vi "7AM.vi"() -> ()   [LabVIEW 2013]
uses:
  <vilib>/measure/NI_MABase.lvlib
panel:
  out "Filtered Signal":dynamicdata(graph)
  in  "sampling info 3":cluster{"Fs":dbl, "#s":dbl}={"Fs"=1000.0, "#s"=1000.0} {"Fs" format="%.2p"}
  in  "ac1":dbl=1.0 format="%0.2p"
  in  "fc1":dbl=10.0 format="%0.2p"
  out "AM Modulared Signal":waveform(dbl)(graph)
  out "carrier signal":waveform(dbl)(graph)
  out "message signal":waveform(dbl)(graph)
  in  "sampling info 2":cluster{"Fs":dbl, "#s":dbl}={"Fs"=1000.0, "#s"=1000.0} {"Fs" format="%.2p"}
  in  "fc":dbl=10.0 format="%0.2p"
  in  "ac":dbl=1.0 format="%0.2p"
  in  "am":dbl=1.0 format="%0.2p"
  in  "fm":dbl=10.0 format="%0.2p"
  in  "sampling info":cluster{"Fs":dbl, "#s":dbl}={"Fs"=1000.0, "#s"=1000.0} {"Fs" format="%.2p"}
  # "23A91A0417\nG SURESH\nECE-A"
  # "Amplitude Modulation Using LabVIEW"
  # "critical Modulation"
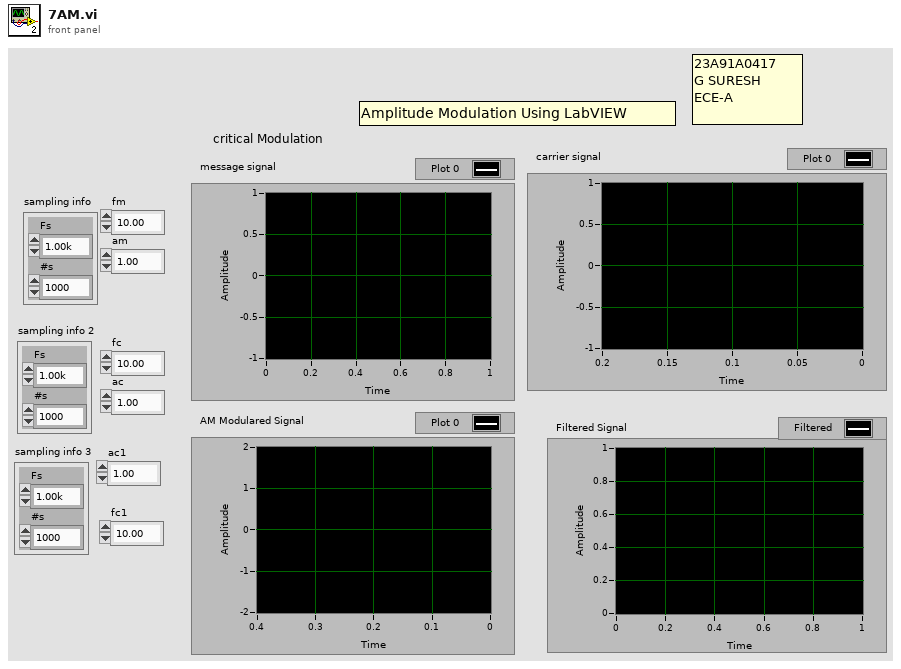
[diagram p1: front panel]
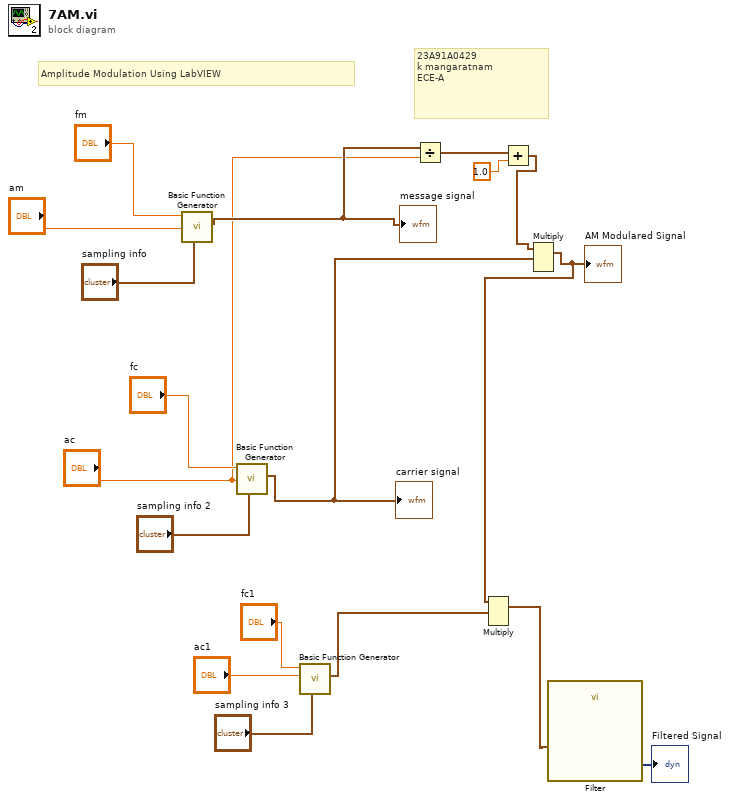
[diagram p0: block diagram]
diagram:
  # "23A91A0429\nk mangaratnam\nECE-A"
  # "Amplitude Modulation Using LabVIEW"
  n1 = call <vilib>:"Basic Function Generator.vi"("sampling info"="sampling info", "amplitude"="am", "frequency"="fm") -> ("signal out"=w2:waveform(dbl))  [unwired: 6 in, 2 out]
  "message signal" <- w2
  n2 = call <vilib>:"Basic Function Generator.vi"("sampling info"="sampling info 2", "amplitude"="ac", "frequency"="fc") -> ("signal out"=w10:waveform(dbl))  [unwired: 6 in, 2 out]
  "carrier signal" <- w10
  n3 = call <vilib>:"Basic Function Generator.vi"("sampling info"="sampling info 3", "amplitude"="ac1", "frequency"="fc1") -> ("signal out"=w6:waveform(dbl))  [unwired: 6 in, 2 out]
  n4 = Divide(x=w2, y="ac") -> (x/y=w13:waveform(dbl))
  n5 = Add(x=w13, y=1.0) -> (x+y=w11:waveform(dbl))
  n6 = Multiply(1:w10, 2:w11) -> (0:w5:waveform(dbl))  [unwired: 1 in, 1 out]
  "AM Modulared Signal" <- w5
  n7 = Multiply(1:w6, 2:w5) -> (0:w4:waveform(dbl))  [unwired: 1 in, 1 out]
  n8 = call "Filter"("Signal"=w4) -> ("Filtered Signal"=→"Filtered Signal":dynamicdata)  [unwired: 9 in, 1 out]
